vi "Lidar Setting.vi"() -> ()   [LabVIEW 2016]
panel:
  in  "Angular resolution 0.25 / 0.5":dbl=0.25
  in  "address":string="192.168.0.204"
  in  "port number":u16=2111
  out "Log in to device":bool
  out "Basic settings":bool
  out "Configure measurement angle":bool
  out "Set to run":bool
  in  "Frequency":u16(ring) items=["25Hz", "50Hz"]
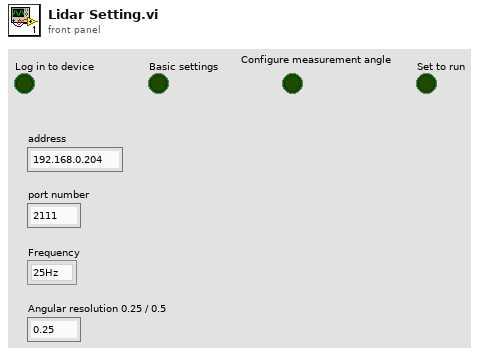
[diagram p1: front panel]
types:
  T1 = enum16{"Standard", "Buffered", "CRLF", "Immediate"}
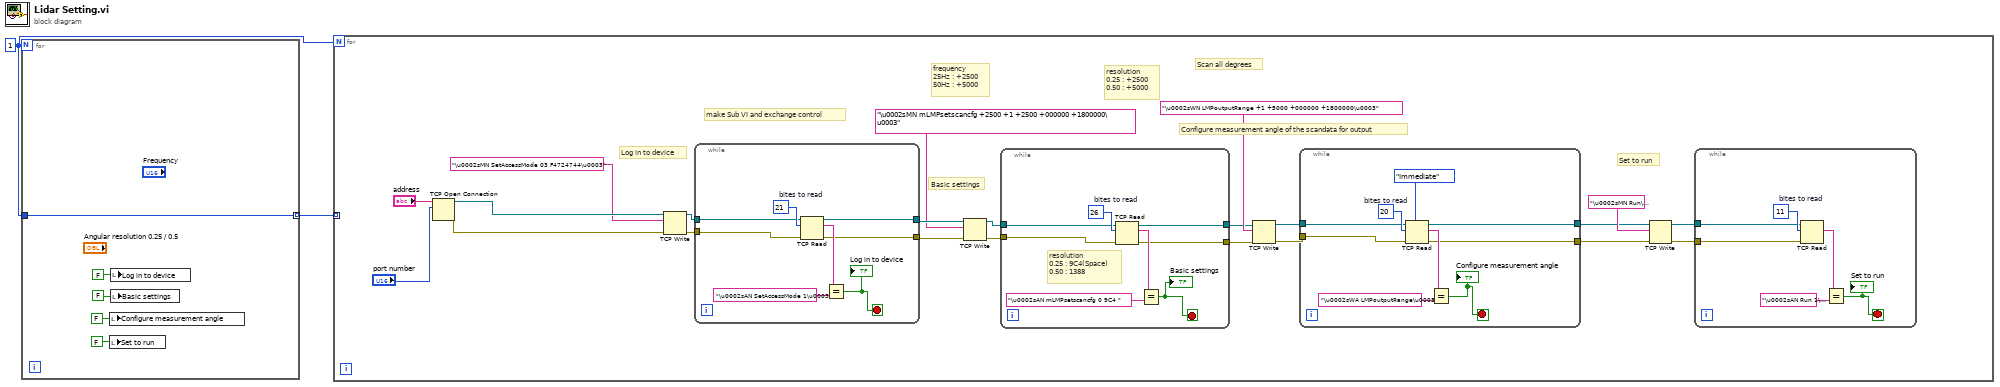
[diagram p0: block diagram]
diagram:
  w1 = 1
  n1 = for {
    N: w1 -> [_]
    tunnel: [w3] -> w2 mode=indexing
    tunnel: w1 -> [w3]
    n2 = local write "Configure measurement angle"(FALSE ("Configure measurement angle")) -> ()
    n3 = local write "Set to run"(FALSE ("Set to run")) -> ()
    n4 = local write "Log in to device"(FALSE ("Log in to device")) -> ()
    n5 = local write "Basic settings"(FALSE ("Basic settings")) -> ()
  }
  n6 = for {
    N: w1 -> [_]
    tunnel: w2 -> [_] mode=indexing
    # "resolution\n0.25 : +2500\n0.50 : +5000"
    # "frequency\n25Hz : +2500\n50Hz : +5000"
    # "Set to run"
    # "Scan all degrees"
    # "Configure measurement angle of the scandata for output"
    # "make Sub VI and exchange control"
    # "Basic settings"
    # "Log in to device"
    n7 = TCP Open Connection(address="address", remote port or service name="port number") -> (connection ID=w26:refnum<k5>, error out=w27:errorcluster)  [unwired: 3 in]
    n8 = TCP Write(connection ID=w26, data in="\u0002sMN SetAccessMode 03 F4724744\u0003" ("데이터 입력"), error in (no error)=w27) -> (connection ID out=w24:refnum<k5>, error out=w25:errorcluster)  [unwired: 1 in, 1 out]
    n9 = while {
      tunnel: w25 -> [w60]
      tunnel: w24 -> [w58]
      tunnel: [w54] -> w22
      tunnel: [w53] -> w20
      stop <- w56 stop-if-true
      w59 = 21  # bites to read
      n10 = TCP Read(connection ID=w58, bytes to read=w59, error in (no error)=w60) -> (connection ID out=w54:refnum<k5>, data out=w57:string, error out=w53:errorcluster)  [unwired: 2 in]
      n11 = Equal?(x=w57, y="\u0002sAN SetAccessMode 1\u0003") -> (x = y?=w56:bool)
      "Log in to device" <- w56
    }
    n12 = TCP Write(connection ID=w22, data in="\u0002sMN mLMPsetscancfg +2500 +1 +2500 +000000 +1800000\u0003" ("데이터 입력"), error in (no error)=w20) -> (connection ID out=w18:refnum<k5>, error out=w19:errorcluster)  [unwired: 1 in, 1 out]
    n13 = while {
      tunnel: w19 -> [w52]
      tunnel: w18 -> [w50]
      tunnel: [w47] -> w13
      tunnel: [w46] -> w14
      stop <- w45 stop-if-true
      w51 = 26  # bites to read
      # "resolution\n0.25 : 9C4(Space)\n0.50 : 1388"
      n14 = TCP Read(connection ID=w50, bytes to read=w51, error in (no error)=w52) -> (connection ID out=w47:refnum<k5>, data out=w49:string, error out=w46:errorcluster)  [unwired: 2 in]
      n15 = Equal?(x=w49, y="\u0002sAN mLMPsetscancfg 0 9C4 ") -> (x = y?=w45:bool)
      "Basic settings" <- w45
    }
    n16 = TCP Write(connection ID=w13, data in="\u0002sWN LMPoutputRange +1 +5000 +000000 +1800000\u0003" ("데이터 입력"), error in (no error)=w14) -> (connection ID out=w17:refnum<k5>, error out=w16:errorcluster)  [unwired: 1 in, 1 out]
    n17 = while {
      tunnel: w16 -> [w44]
      tunnel: w17 -> [w42]
      tunnel: [w38] -> w9
      tunnel: [w37] -> w8
      stop <- w40 stop-if-true
      w43 = 20  # bites to read
      n18 = TCP Read(connection ID=w42, bytes to read=w43, error in (no error)=w44, 7:T1."Immediate" ("모드(standard)")) -> (connection ID out=w38:refnum<k5>, data out=w41:string, error out=w37:errorcluster)  [unwired: 1 in]
      n19 = Equal?(x=w41, y="\u0002sWA LMPoutputRange\u0003") -> (x = y?=w40:bool)
      "Configure measurement angle" <- w40
    }
    n20 = TCP Write(connection ID=w9, data in="\u0002sMN Run\u0003" ("데이터 입력"), error in (no error)=w8) -> (connection ID out=w10:refnum<k5>, error out=w11:errorcluster)  [unwired: 1 in, 1 out]
    n21 = while {
      tunnel: w11 -> [w35]
      tunnel: w10 -> [w33]
      stop <- w31 stop-if-true
      w34 = 11  # bites to read
      n22 = TCP Read(connection ID=w33, bytes to read=w34, error in (no error)=w35) -> (data out=w32:string)  [unwired: 2 in, 2 out]
      n23 = Equal?(x=w32, y="\u0002sAN Run 1\u0003") -> (x = y?=w31:bool)
      "Set to run" <- w31
    }
  }
